vi "King Swap 2.vi"(0 "1D Board":T2[](array[typedef]), 5 "DT Team #":i32, 11 "error in (no error)":errorcluster) -> (4 "1D Board Out":T2[](array[typedef]), 6 "Cell to move to":i32, 8 "Output Text":string, 15 "error out":errorcluster)   [LabVIEW 2014]
uses:
  Typedefs/Board Cell.ctl
  Typedefs/Cell Occupancy.ctl
  Typedefs/Select Empty DT or Both.ctl
  Dragon Tamers.lvlib
panel:
  in  "Enum":T1=enum."Empty and DT"
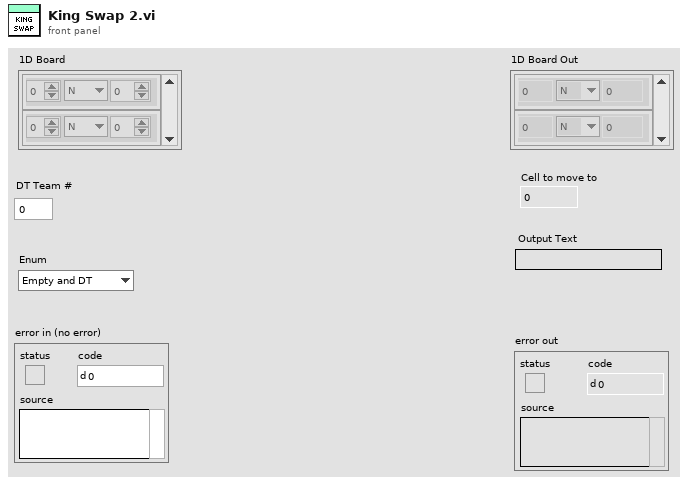
[diagram p1: front panel]
types:
  T1 = typedef "Select Empty DT or Both.ctl" = enum16{"Empty Only", "DT Cells Only", "Empty and DT"}
  T2 = typedef "Dragon Tamers.lvlib/Board Cell.ctl" = cluster{"Team":i32, "Occu.":T3, "Count":i32}
  T3 = typedef "Dragon Tamers.lvlib/Cell Occupancy.ctl" = enum16{"N", "C", "K"}
  T4 = typedef "Dragon Tamers.lvlib/Parsed Board.ctl" = cluster{"DT King":i32, "Opp King":i32, "Count":i32[], "Empty Cells":i32[], "DT Cells":i32[], "Opp Cells":i32[], "DT Team":i32, "Opp. Team":i32}
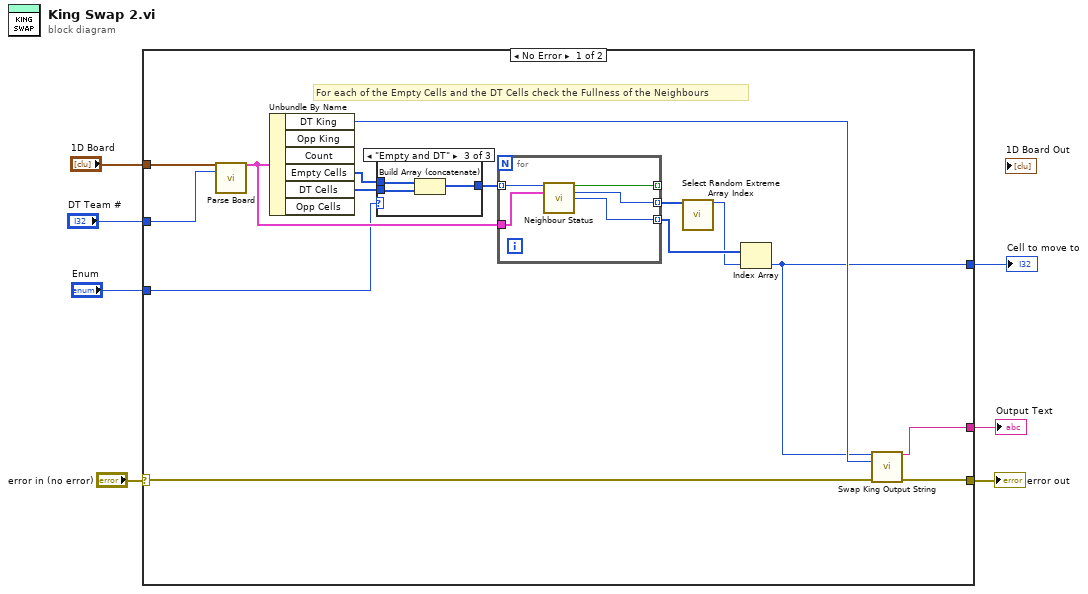
[diagram p0: block diagram]
diagram:
  n1 = case shown="No Error" "error in (no error)" {
    selector: "error in (no error)" -> [w14 w33]
    tunnel: [w20 w33] -> w6
    tunnel: "1D Board" -> [w22 _]
    tunnel: "DT Team #" -> [w21 _]
    tunnel: [w13 _] -> w3
    tunnel: "Enum" -> [w9 _]
    tunnel: [w8 _] -> w1
    frame No Error {
      # "For each of the Empty Cells and the DT Cells check the Fullness of the Neighbours"
      n2 = call "Parse Board.vi"("Board Array"=w22, "DT Team #"=w21) -> ("Parsed Board Info"=w16:T4)  [unwired: 12 in, 1 out]
      n3 = Unbundle By Name(w16) -> ("DT King"=w15:i32, "Empty Cells"=w19:i32[], "DT Cells"=w18:i32[])  [unwired: 3 out]
      n4 = case shown="\"Empty and DT\"" w9 {
        tunnel: w19 -> [w23 _ w27]
        tunnel: w18 -> [_ w24 w26]
        tunnel: [w23 w24 w25] -> w17
        frame "Empty Only", Default {
        }
        frame "DT Cells Only" {
        }
        frame "Empty and DT" {
          n5 = Build Array (concatenate)(w27, w26) -> (w25:i32[])
        }
      }
      n6 = for {
        tunnel: w17 -> [w31] mode=indexing
        tunnel: w16 -> [w32]
        tunnel: [w30] -> _ mode=indexing
        tunnel: [w29] -> w12 mode=indexing
        tunnel: [w28] -> w11 mode=indexing
        n7 = call "Neighbour Status.vi"("Cell"=w31, "Parsed Board"=w32) -> ("Full?"=w30:bool, "Min Count to Max"=w29:i32, "Cell Index"=w28:i32)  [unwired: 10 in, 1 out]
      }
      n8 = call "Select Random Extreme Array Index.vi"("Array"=w12) -> ("Chosen Max Index"=w10:i32)  [unwired: 14 in, 4 out]
      n9 = Index Array(array=w11, index=w10) -> (element=w8:i32)
      n10 = call "Swap King Output String.vi"("New Cell Index"=w8, "Old Cell Index"=w15, "error in (no error)"=w14) -> ("Output Text"=w13:string, "error out"=w20:errorcluster)  [unwired: 11 in]
    }
    frame Error {
    }
  }
  "error out" <- w6
  "Output Text" <- w3
  "Cell to move to" <- w1
